vi "PicTake.vi"() -> ()   [LabVIEW 2016]
uses:
  <vilib>/userdefined/High Color/IMAQdx.ctl
  <vilib>/vision/driver/NI_Vision_Acquisition_Software.lvlib
panel:
  in  "stop":bool
  in  "name(dir in Windows\\Pictures)":string
  out "Image":T1(plugin-control)
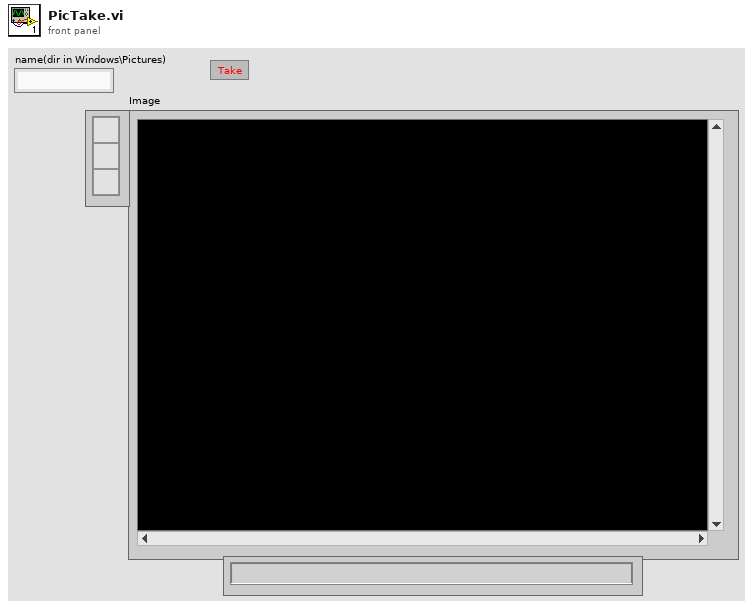
[diagram p1: front panel]
types:
  T1 = typedef "IMAQ Image.ctl" = refnum<image>
  T2 = typedef "IMAQdx.ctl" = refnum<k21>
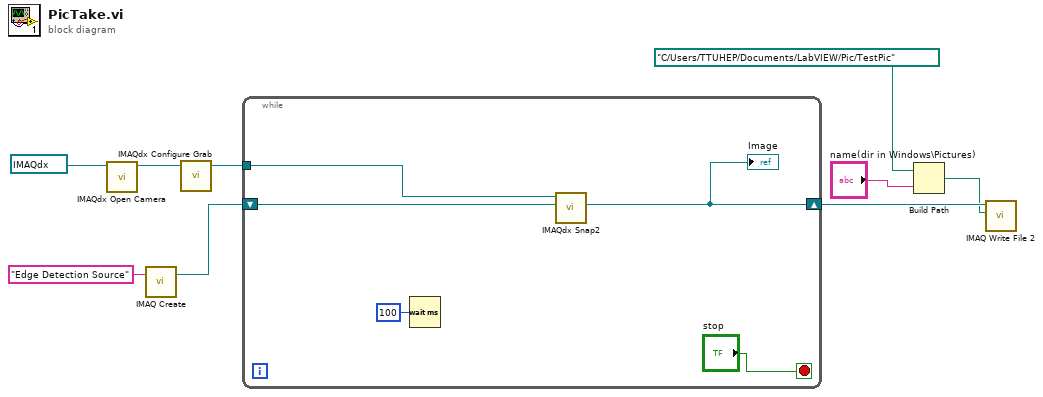
[diagram p0: block diagram]
diagram:
  n1 = call <vilib>:"IMAQdx Open Camera.vi"("Session In"=T2 "cam0") -> ("Session Out"=w8:T2)  [unwired: 9 in, 1 out]
  n2 = call "IMAQ Create"("Image Name"="Edge Detection Source") -> ("New Image"=w5:T1)  [unwired: 4 in, 1 out]
  n3 = call <vilib>:"IMAQdx Configure Grab.vi"("Session In"=w8) -> ("Session Out"=w7:T2)  [unwired: 9 in, 1 out]
  n4 = while {
    tunnel: w7 -> [w14]
    shift-right: [w11] -> w4
    shift-left: w5 -> [w13]
    stop <- "stop" stop-if-true
    n5 = Wait (ms)(milliseconds to wait=u32 100) -> ()  [unwired: 1 out]
    n6 = call <vilib>:"IMAQdx Snap2.vi"("Image In"=w13, "Session In"=w14) -> ("Image Out"=w11:T1)  [unwired: 7 in, 2 out]
    "Image" <- w11
  }
  n7 = Build Path(base path=path "C:/Users/TTUHEP/Documents/LabVIEW/Pic/TestPic", name or relative path="name(dir in Windows\\Pictures)") -> (appended path=w3:path)
  n8 = call-poly "IMAQ Write File 2"("File Path"=w3, "Image"=w4) -> ()  [unwired: 8 in, 2 out]
